vi "Global IP address server.vi"() -> ()   [LabVIEW 2019]
panel:
  in  "ip address pc server":string
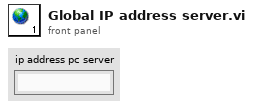
[diagram p1: front panel]
diagram:
